vi "Flatten Wire.vi"(6 "Variant in":variant, 7 "Shift Pressed?":bool, 8 "error in (no error)":errorcluster, 10 "QD Combo Box Ref":refnum<vi>, 11 "QD Launch VI Ref":refnum<vi>) -> (0 "error out":errorcluster, 4 "Variant out":variant)   [LabVIEW 2017]
doc: "If the selected wire has two endpoints, this plugin flattens it by moving one of it endpoints, and moves whatever is connected to the endpoint that was moved. By default, it moves the right endpoint of the wire up or down to be inline with the left endpoint. If the selected wire has more than two endpoints, this plugin does nothing.\n\nIf shift is also pressed, it moves the left endpoint of the wire instead of the right one.\n\nIf multiple wires are selected, it will flatten them in the order that they were selected.\n\nDefault Shortcut - [F]"
uses:
  <vilib>/ErrorRing/Error Ring.xnode
panel:
  in  "Undo Name":string="Quick Drop Keyboard Shortcut"
  # "Do not change the connector pane of this VI.\n\nSee the block diagram for directions on how to use this template."
  # "Specify the name of the Undo transaction"
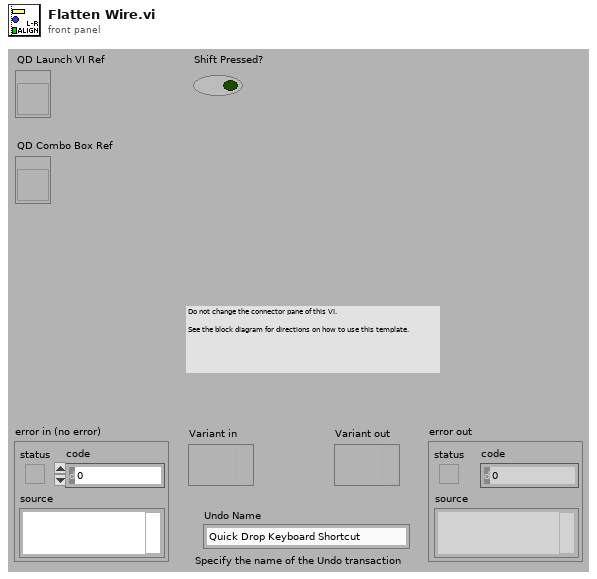
[diagram p1: front panel]
types:
  T1 = enum32{"LooseEnd", "Endpoint", "Bend", "Junction"}
  T2 = cluster{"Position":cluster{"h":i16, "v":i16}, "Flags":i32, "Type":enum32{"LooseEnd", "Endpoint", "Bend", "Junction"}, "Up Joint Index":i16, "Down Joint Index":i16, "Left Joint Index":i16, "Right Joint Index":i16}[]
  T3 = typedef "LVPositionTypeDef.ctl" = cluster{"Left":i32, "Top":i32}
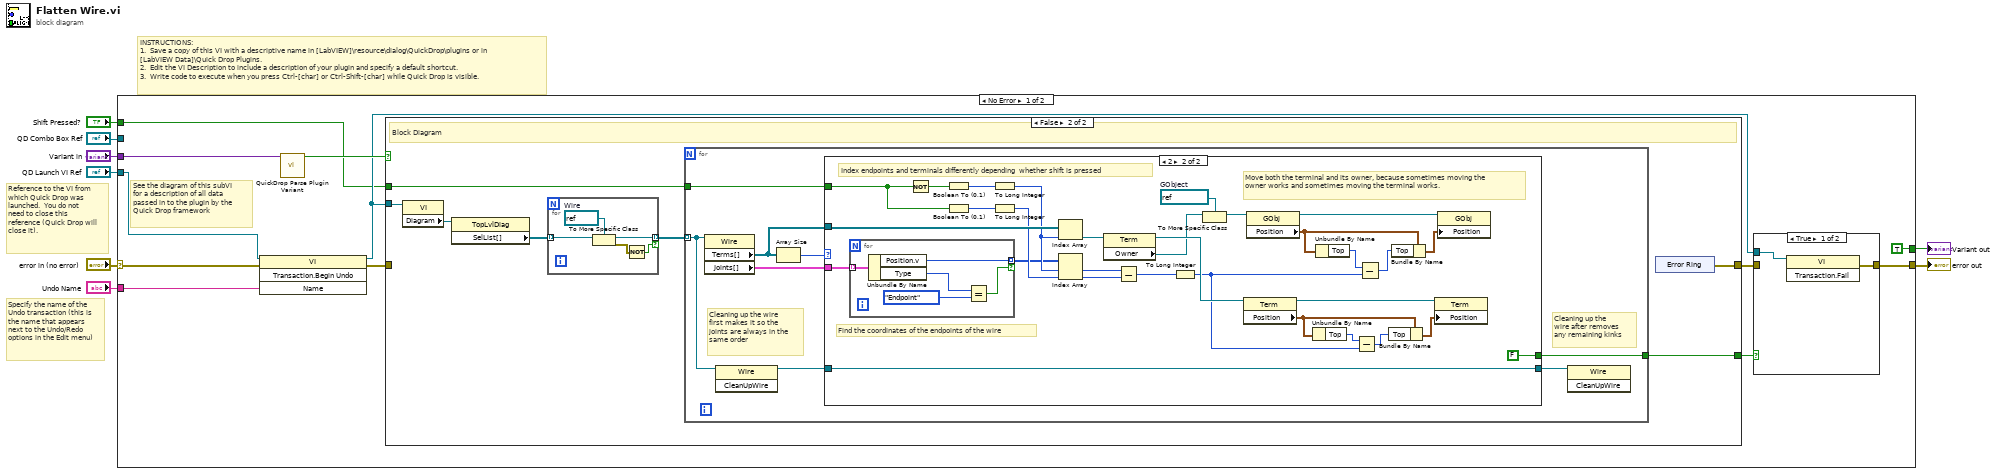
[diagram p0: block diagram]
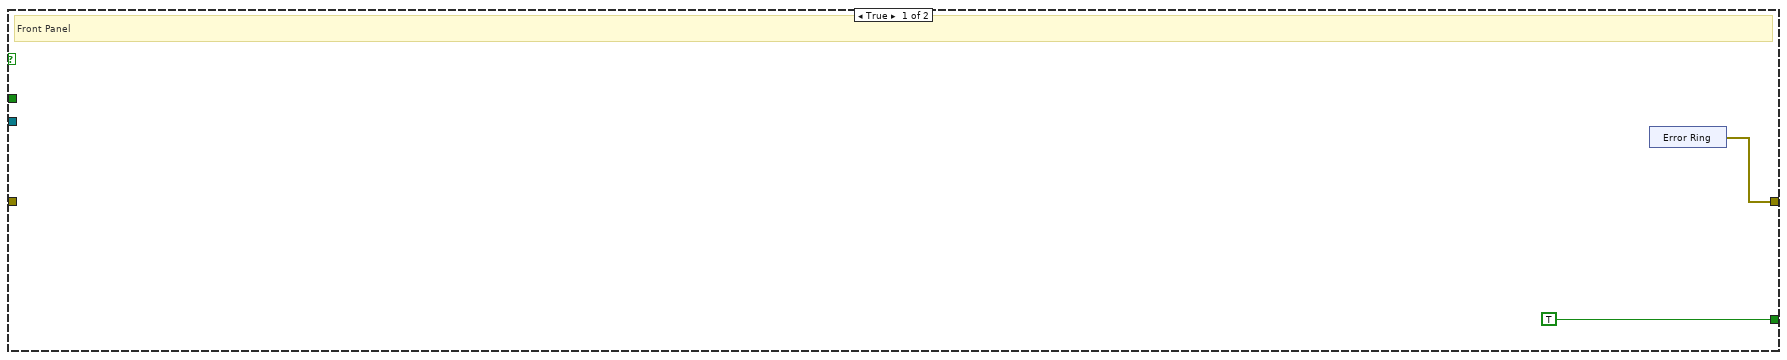
[diagram p2: hidden frame]
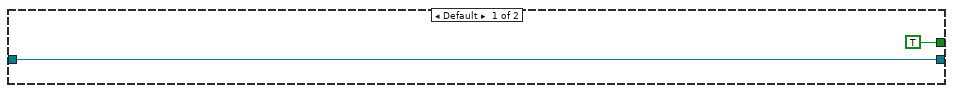
[diagram p3: hidden frame]
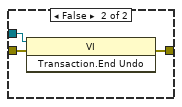
[diagram p4: hidden frame]
diagram:
  # "Specify the name of the Undo transaction (this is the name that appears next to the Undo/Redo options in the Edit menu)"
  # "Reference to the VI from which Quick Drop was launched.  You do not need to close this reference (Quick Drop will close it)."
  # "INSTRUCTIONS:\n1.  Save a copy of this VI with a descriptive name in [LabVIEW]\\resource\\dialog\\QuickDrop\\plugins or in [LabVIEW Data]\\Quick Drop Plugins.\n2.  Edit the VI Description to include a description of your plugin and specify a default shortcut. \n3.  Write code to execute when you press Ctrl-[char] or Ctrl-Shift-[char] while Quick Drop is visible."
  n1 = case shown="No Error" "error in (no error)" {
    selector: "error in (no error)" -> [w19 w87]
    tunnel: [w14 w87] -> w7
    tunnel: "QD Launch VI Ref" -> [w18 _]
    tunnel: "Shift Pressed?" -> [w11 _]
    tunnel: "QD Combo Box Ref" -> [_ _]
    tunnel: "Variant in" -> [w20 _]
    tunnel: "Undo Name" -> [w17 _]
    tunnel: [TRUE _] -> w1
    frame No Error {
      # "See the diagram of this subVI for a description of all data passed in to the plugin by the Quick Drop framework"
      n2 = invoke class="VI" method="Transaction.Begin Undo"(reference=w18, error in=w19, "Name"=w17) -> (reference out=w13:refnum<vi>, error out=w12:errorcluster)  [unwired: 1 in, 2 out]
      n3 = call <vilib>:"QuickDrop Parse Plugin Variant.vi"("QDKS Variant in"=w20) -> ("QD Launch VI Panel?"=w15:bool)  [unwired: 12 in, 2 out]
      n4 = case shown="False" w15 {
        tunnel: w12 -> [_ _]
        tunnel: w13 -> [_ w29]
        tunnel: w11 -> [_ w27]
        tunnel: [w22 w30] -> w10
        tunnel: [TRUE w26] -> w9
        frame True {
          # "Front Panel"
          n5 = xnode "Error Ring"() -> ("error out"=w22:errorcluster)
        }
        frame False {
          # "Block Diagram"
          n6 = property class="VI"(reference=w29) -> ("Diagram"=w28:refnum<vi>)  [unwired: 1 in, 2 out]
          n7 = property class="TopLvlDiag"(reference=w28) -> ("SelList[]"=w25:refnum<vi>[])  [unwired: 1 in, 2 out]
          n8 = for {
            tunnel: w25 -> [w35] mode=indexing
            tunnel: [w33] -> w24 mode=indexing if=w31
            w34 = refnum<vi> refnum  # Wire
            n9 = To More Specific Class(target class=w34, reference=w35) -> (specific class reference=w33:refnum<vi>, error out=w32:errorcluster)  [unwired: 1 in]
            n10 = Not(x=w32) -> (.not. x?=w31:bool)
          }
          n11 = for {
            tunnel: w27 -> [w40]
            tunnel: w24 -> [w38] mode=indexing
            tunnel: [w42] -> w26
            # "Cleaning up the\nwire after removes\nany remaining kinks"
            # "Cleaning up the wire\nfirst makes it so the\njoints are always in the \nsame order"
            n12 = property class="Wire"(reference=w38) -> ("Terms[]"=w39:refnum<vi>[], "Joints[]"=w41:T2)  [unwired: 1 in, 2 out]
            n13 = invoke class="Wire" method="CleanUpWire"(reference=w38) -> (reference out=w37:refnum<vi>)  [unwired: 2 in, 2 out]
            n14 = Array Size(array=w39) -> (size(s)=w43:i32)
            n15 = case shown="2" w43 {
              tunnel: [TRUE FALSE] -> w42
              tunnel: w41 -> [_ w74]
              tunnel: w40 -> [_ w72]
              tunnel: w39 -> [_ w69]
              tunnel: w37 -> [w44 w46]
              tunnel: [w44 w46] -> w36
              frame Default {
              }
              frame 2 {
                w48 = refnum<vi> refnum  # GObject
                # "Index endpoints and terminals differently depending  whether shift is pressed"
                # "Find the coordinates of the endpoints of the wire"
                # "Move both the terminal and its owner, because sometimes moving the owner works and sometimes moving the terminal works."
                n16 = for {
                  tunnel: w74 -> [w79] mode=indexing
                  tunnel: [w76] -> w47 mode=indexing if=w77
                  n17 = Unbundle By Name(w79) -> ("Position.v"=w76:i16, "Type"=w78:T1)
                  n18 = Equal?(x=w78, y=T1."Endpoint") -> (x = y?=w77:bool)
                }
                n19 = Not(x=w72) -> (.not. x?=w73:bool)
                n20 = Boolean To (0,1)(Boolean=w73) -> (0, 1=w71:i16)
                n21 = Boolean To (0,1)(Boolean=w72) -> (0, 1=w70:i16)
                n22 = To Long Integer(number=w71) -> (32bit integer=w68:i32)
                n23 = To Long Integer(number=w70) -> (32bit integer=w49:i32)
                n24 = Index Array(array=w69, index=w68) -> (element=w65:refnum<vi>)
                n25 = Index Array(array=w47, index #1=w68, index #2=w49) -> (element #1=w67:i16, element #2=w66:i16)
                n26 = property class="Term"(reference=w65) -> (reference out=w63:refnum<vi>, "Owner"=w50:refnum<vi>)  [unwired: 1 in, 1 out]
                n27 = Subtract(x=w67, y=w66) -> (x-y=w64:i16)
                n28 = To Long Integer(number=w64) -> (32bit integer=w62:i32)
                n29 = To More Specific Class(target class=w48, reference=w50) -> (specific class reference=w51:refnum<vi>)  [unwired: 1 in, 1 out]
                n30 = property class="Term"(reference=w63) -> (reference out=w57:refnum<vi>, "Position"=w59:T3)  [unwired: 1 in, 1 out]
                n31 = property class="GObj"(reference=w51) -> (reference out=w55:refnum<vi>, "Position"=w53:T3)  [unwired: 1 in, 1 out]
                n32 = Unbundle By Name(w59) -> ("Top"=w60:i32)
                n33 = Unbundle By Name(w53) -> ("Top"=w52:i32)
                n34 = Subtract(x=w60, y=w62) -> (x-y=w61:i32)
                n35 = Subtract(x=w52, y=w62) -> (x-y=w56:i32)
                n36 = Bundle By Name(cluster=w59, "Top"=w61) -> (w58:T3)
                n37 = Bundle By Name(cluster=w53, "Top"=w56) -> (w54:T3)
                n38 = property class="Term"(reference=w57, "Position"=w58) -> ()  [unwired: 1 in, 2 out]
                n39 = property class="GObj"(reference=w55, "Position"=w54) -> ()  [unwired: 1 in, 2 out]
              }
            }
            n40 = invoke class="Wire" method="CleanUpWire"(reference=w36) -> ()  [unwired: 2 in, 3 out]
          }
          n41 = xnode "Error Ring"() -> ("error out"=w30:errorcluster)
        }
      }
      n42 = case shown="True" w9 {
        tunnel: w13 -> [w82 w85]
        tunnel: [w83 w86] -> w14
        tunnel: w10 -> [_ w84]
        frame True {
          n43 = invoke class="VI" method="Transaction.Fail"(reference=w82) -> (error out=w83:errorcluster)  [unwired: 2 in, 2 out]
        }
        frame False {
          n44 = invoke class="VI" method="Transaction.End Undo"(reference=w85, error in=w84) -> (error out=w86:errorcluster)  [unwired: 1 in, 2 out]
        }
      }
    }
    frame Error {
    }
  }
  "error out" <- w7
  "Variant out" <- w1
